vi "Station_V3.0_Test.vi"() -> ()   [LabVIEW 2023]
panel:
  in  "로그기록_버튼 2":bool
  in  "관리자_버튼 3":bool
  in  "관리자_버튼 2":bool
  in  "탭 컨트롤":enum32{"음향 측정 데이터", "TMC Set 데이터", "유속데이터"}(tab)
  out "RX_LED":bool
  out "TX_LED":bool
  out "RX_LED":bool
  out "TX_LED":bool
  out "TMC_SET_3":dbl[](graph)
  out "TMC_SET_2":dbl[](graph)
  in  "여러 열 리스트박스 2":i32(listbox)
  in  "여러 열 리스트박스":i32(listbox)
  out "로그기록":string
  out "평균 음속 데이터":dbl(graph)
  out "유속 데이터":dbl(graph)
  in  "로그기록_버튼":bool
  in  "관리자_버튼":bool
  in  "측정 그래프_버튼":bool
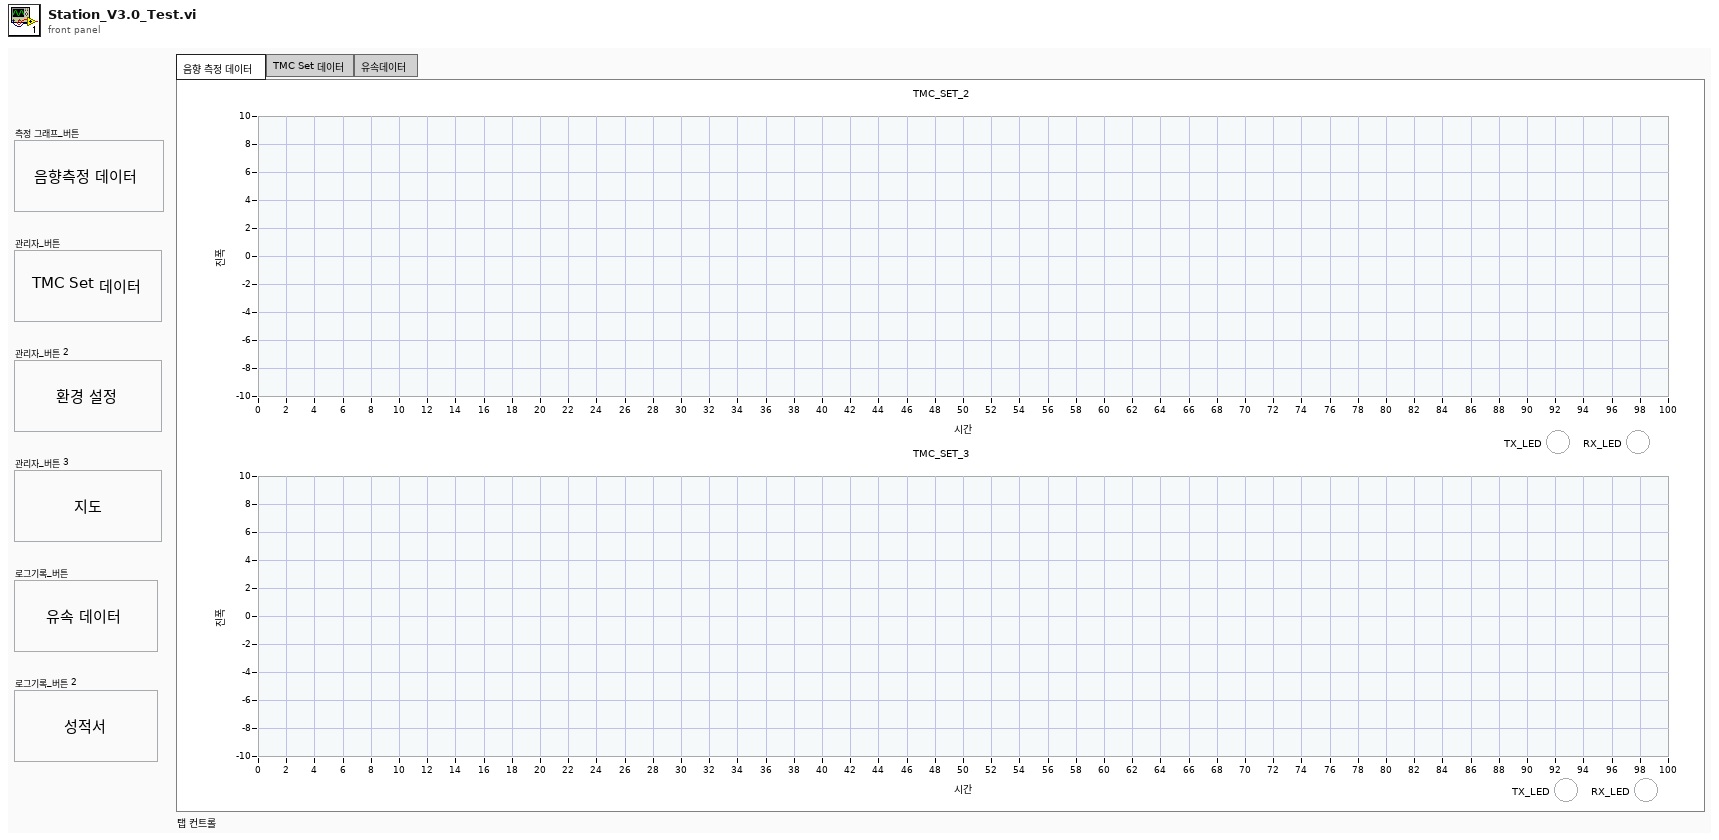
[diagram p1: front panel]
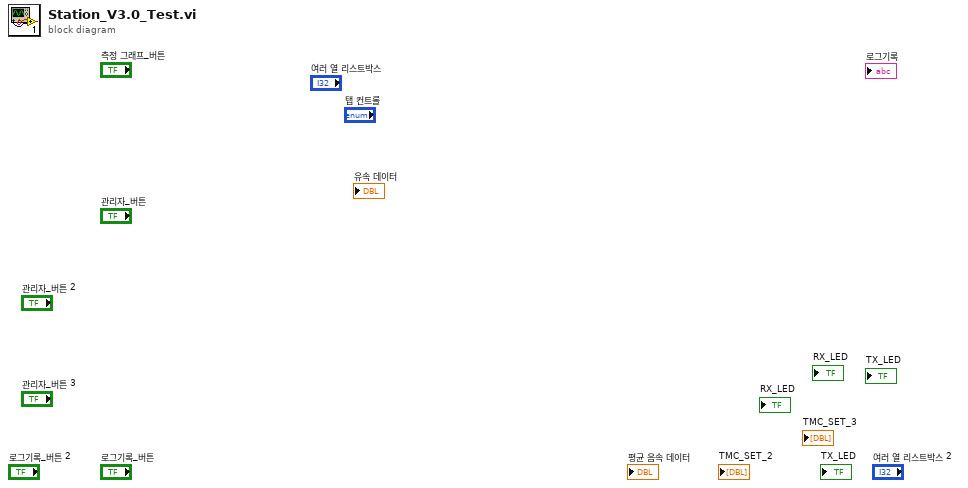
[diagram p0: block diagram]
diagram:
